vi "Read Message.vi"(11 "IAction in":refnum<class "IAction.lvclass">) -> (2 "Message":string, 3 "IAction out":refnum<class "IAction.lvclass">)   [LabVIEW 2019, in "IAction.lvclass"]
uses:
  IAction.lvclass
  IAction.lvclass/IAction.ctl
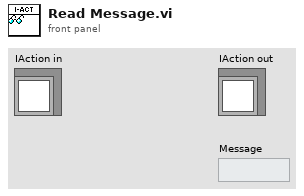
[diagram p1: front panel]
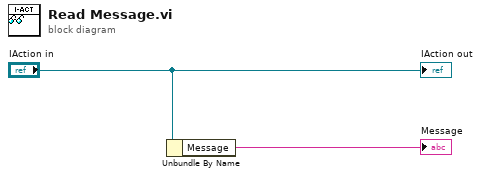
[diagram p0: block diagram]
diagram:
  n1 = Unbundle By Name("IAction in") -> ("Message"=→"Message":string)
  "IAction out" <- "IAction in"
